vi "AIScaleAndLimit.vi"(0 "UnscaledAI":i16[](array[numeric])=[0, 0, 0, 0, 0, 0, 0, 0, 0, 0, 0, 0, 0, 0, 0, 0], 1 "ConfigRegisters":T2, 2 "LimitsRegisters":T1={"HighLimits"="HighLimits", "LowLimits"="LowLimits", "ClearLimits"="ClearLimits", "LimitsFlag"="ClearLimits"}, 9 "input valid":bool=TRUE) -> (4 "ScaledAI":sgl[](array[numeric]), 6 "HighLimits":u16, 8 "LowLimits":u16, 10 "ready for input":bool, 14 "LimitsFlag":bool, 15 "output valid":bool)   [LabVIEW 2017, in "ScaleAndLimit.lvlib"]
doc: "Main FPGA IP Block to scale U32 datatypes to SGL and check for limits."
uses:
  ScaleAndLimit.lvlib
  ConfigRegisters.ctl
  LimitsRegisters.ctl
  <vilib>/rvi/DataTransferAndStorage/Container/Common/niFpgaContainerExecOnDevCompGetState.vi
  <vilib>/rvi/Emulation/niFpgaEmulationIsFPGAContextNoSignature.vi
  <vilib>/rvi/DataTransferAndStorage/Container/Common/niFpgaContainerGetUniqueNameForEmu.vi
  <vilib>/rvi/Memory/Memory_Emulation/niFpgaMemoryEmulationCacheClearOnFirstRun.vi
  <vilib>/rvi/Memory/Memory_Emulation/nirvimemoryEmulationManagerCache_MakeExclusive.vi
  <vilib>/rvi/Memory/Memory_Emulation/niFpgaMemoryEmulationValidateCache.vi
  <vilib>/rvi/Memory/Memory_Emulation/nirvimemoryEmulationManagerCache_InsertValue.vi
  <vilib>/Utility/error.llb/Clear Errors.vi
  <vilib>/rvi/Memory/Memory_Emulation/nirvimemoryEmulationManagerCache_ReleaseExclusive.vi
  <vilib>/rvi/Memory/Memory_Emulation/nirvimemoryEmulationManagerCache_GetValue.vi
  <vilib>/rvi/Memory/Memory_Emulation/nirvimemoryEmulationManagerCache_SetValue.vi
  <vilib>/rvi/Emulation/niFpgaProcessEmulError.vi
  <vilib>/rvi/Emulation/niFpgaSctlEmulationGetInTimedLoop.vi
  <vilib>/rvi/DataTransferAndStorage/Container/XNode/niFpgaContainer.xnode
  <vilib>/rvi/DataTransferAndStorage/Register/Emulation/niFpgaRegisterEmulationRefIn.vi
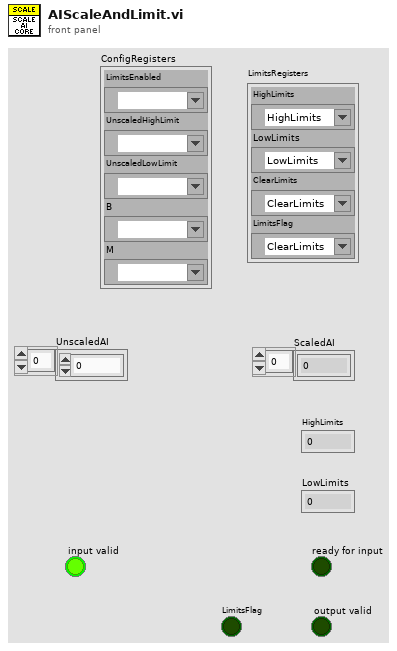
[diagram p1: front panel]
types:
  T1 = typedef "ScaleAndLimit.lvlib/LimitsRegisters.ctl" = cluster{"HighLimits":refnum<k21>, "LowLimits":refnum<k21>, "ClearLimits":refnum<k21>, "LimitsFlag":refnum<k21>}
  T2 = typedef "ScaleAndLimit.lvlib/ConfigRegisters.ctl" = cluster{"LimitsEnabled":refnum<k21>, "UnscaledHighLimit":refnum<k21>, "UnscaledLowLimit":refnum<k21>, "B":refnum<k21>, "M":refnum<k21>}
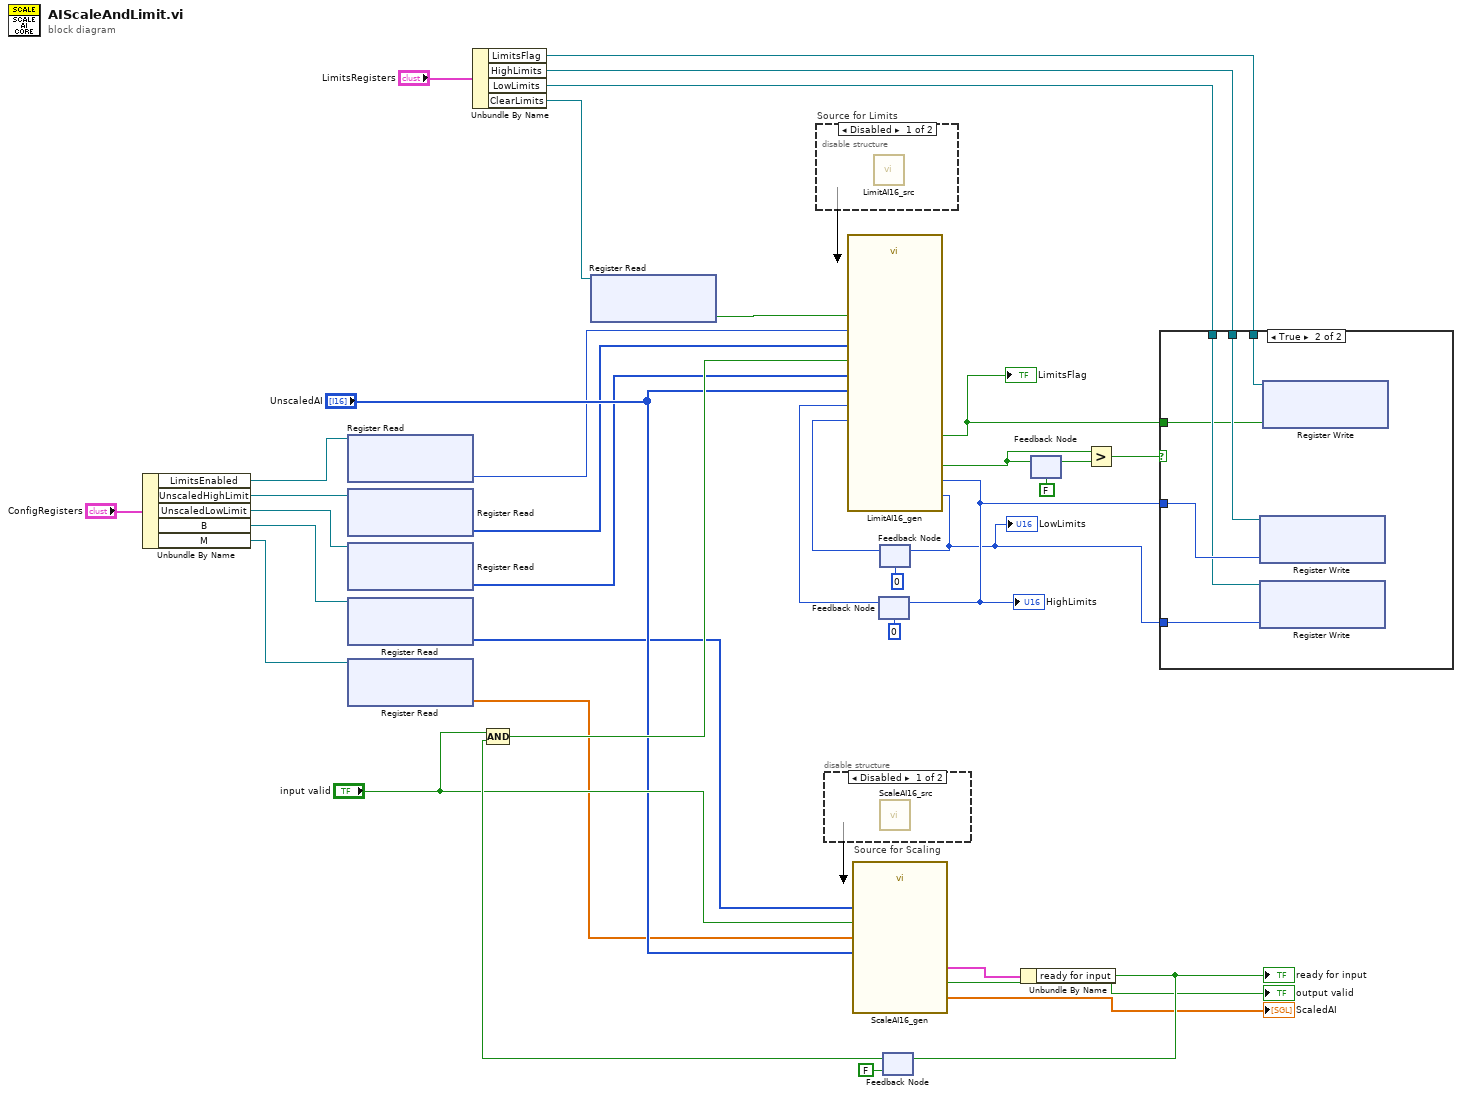
[diagram p0: block diagram]
diagram:
  n1 = Unbundle By Name("ConfigRegisters") -> ("LimitsEnabled"=w20:refnum<k21>, "UnscaledHighLimit"=w18:refnum<k21>, "UnscaledLowLimit"=w16:refnum<k21>, "B"=w14:refnum<k21>, "M"=w12:refnum<k21>)
  n2 = xnode ("Register Read")("Register In"=w20) -> ("Data"=w19:u16)  [unwired: 1 out]
  n3 = xnode ("Register Read")("Register In"=w18) -> ("Data"=w17:i16[])  [unwired: 1 out]
  n4 = xnode ("Register Read")("Register In"=w16) -> ("Data"=w15:i16[])  [unwired: 1 out]
  n5 = xnode ("Register Read")("Register In"=w14) -> ("Data"=w13:i16[])  [unwired: 1 out]
  n6 = xnode ("Register Read")("Register In"=w12) -> ("Data"=w11:sgl[])  [unwired: 1 out]
  n7 = Unbundle By Name("LimitsRegisters") -> ("LimitsFlag"=w4:refnum<k21>, "HighLimits"=w8:refnum<k21>, "LowLimits"=w7:refnum<k21>, "ClearLimits"=w2:refnum<k21>)
  n8 = xnode ("Register Read")("Register In"=w2) -> ("Data"=w1:bool)  [unwired: 1 out]
  n9 = disable-structure "Source for Limits" shown="Disabled" {
    frame Disabled {
      n10 = call "LimitAI16_src.vi"() -> ()  [unwired: 13 in, 3 out]
    }
    frame Enabled {
    }
  }
  n11 = disable-structure "Source for Scaling" shown="Disabled" {
    frame Disabled {
      n12 = call "ScaleAI16_src.vi"() -> ()  [unwired: 15 in, 1 out]
    }
    frame Enabled {
    }
  }
  n13 = call "ScaleAI16_gen.vi"("M"=w11, "B"=w13, "UnscaledAI"="UnscaledAI", "input valid"="input valid") -> ("ScaledAI"=→"ScaledAI":sgl[], "output valid"=→"output valid":bool, "feedback signals"=w24:cluster{"ready for input":bool})  [unwired: 9 in]
  n14 = feedback #1(u16 0 ("RawAIFaultHighOut")) -> (w37:u16)
  n15 = feedback #2(u16 0 ("RawAIFaultLowOut")) -> (w36:u16)
  n16 = feedback #3(FALSE ("ready for input")) -> (w29:bool)
  n17 = Compound Arithmetic op=AND("input valid", w29) -> (w28:bool)
  n18 = call "LimitAI16_gen.vi"("ClearLimit"=w1, "HighLimit"=w17, "UnscaledAI"="UnscaledAI", "UnscaledLimitLowIn"=w36, "UnscaledLimitHighIn"=w37, "input valid"=w28, "LowLimit"=w15, "LimitiEnabled"=w19) -> ("UnscaledLimitLowOut"=w5:u16, "UnscaledLimitHighOut"=w6:u16, "LimitReached"=w3:bool, "output valid"=w31:bool)  [unwired: 3 in, 1 out]
  "LimitsFlag" <- w3
  "HighLimits" <- w6
  "LowLimits" <- w5
  n19 = feedback-in #1(w6) -> ()
  n20 = feedback-in #2(w5) -> ()
  n21 = Unbundle By Name(w24) -> ("ready for input"=w30:bool)
  "ready for input" <- w30
  n22 = feedback-in #3(w30) -> ()
  n23 = feedback-in #4(w31) -> ()
  n24 = feedback #4(FALSE ("faulted")) -> (w32:bool)
  n25 = Greater?(x=w31, y=w32) -> (0:w9:bool)
  n26 = case shown="True" w9 {
    tunnel: w8 -> [_ w43]
    tunnel: w7 -> [_ w41]
    tunnel: w6 -> [_ w42]
    tunnel: w5 -> [_ w40]
    tunnel: w4 -> [_ w39]
    tunnel: w3 -> [_ w38]
    frame False {
    }
    frame True {
      n27 = xnode ("Register Write")("Data"=w42, "Register In"=w43) -> ()  [unwired: 1 out]
      n28 = xnode ("Register Write")("Data"=w40, "Register In"=w41) -> ()  [unwired: 1 out]
      n29 = xnode ("Register Write")("Data"=w38, "Register In"=w39) -> ()  [unwired: 1 out]
    }
  }
